vi "MARS Scan Data Analysis Wrapper.vi"(9 "Ratio Graph in":refnum<vi>, 10 "Listbox":i32[](array[numeric]), 11 "Active Meas.":i32) -> (0 "FoM Graph":dbl[][](array[numeric]), 1 "Fit Histogram":i32[][](array[numeric]), 2 "Ratio Graph":i32[][](array[numeric]), 3 "FoM":dbl, 4 "FoM_2nd_max":dbl, 5 "FoM_1st_max":dbl, 6 "FoM_2nd_min":dbl, 7 "FoM_1st_min":dbl)   [LabVIEW 2015]
uses:
  Data_Analysis_subvis/MARS_Scan_Data_Analysis_global.vi
panel:
  out "2nd period 2":dbl[](array[numeric])
  out "1st period 2":dbl[](array[numeric])
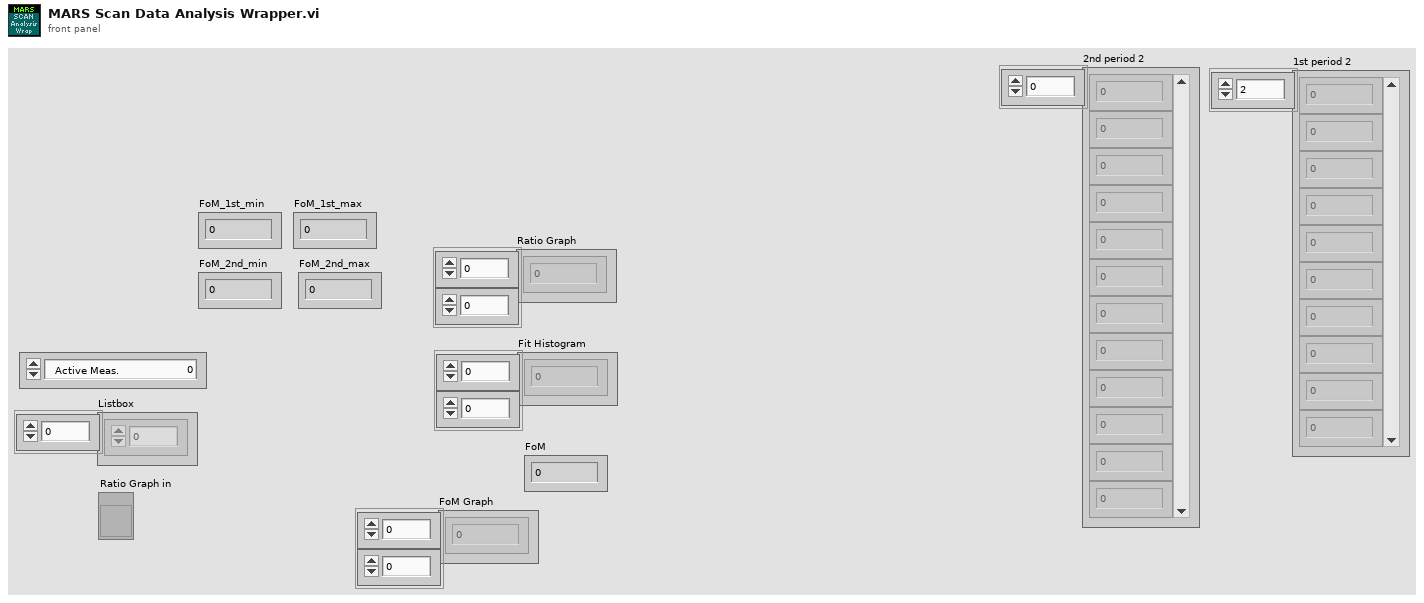
[diagram p1: front panel]
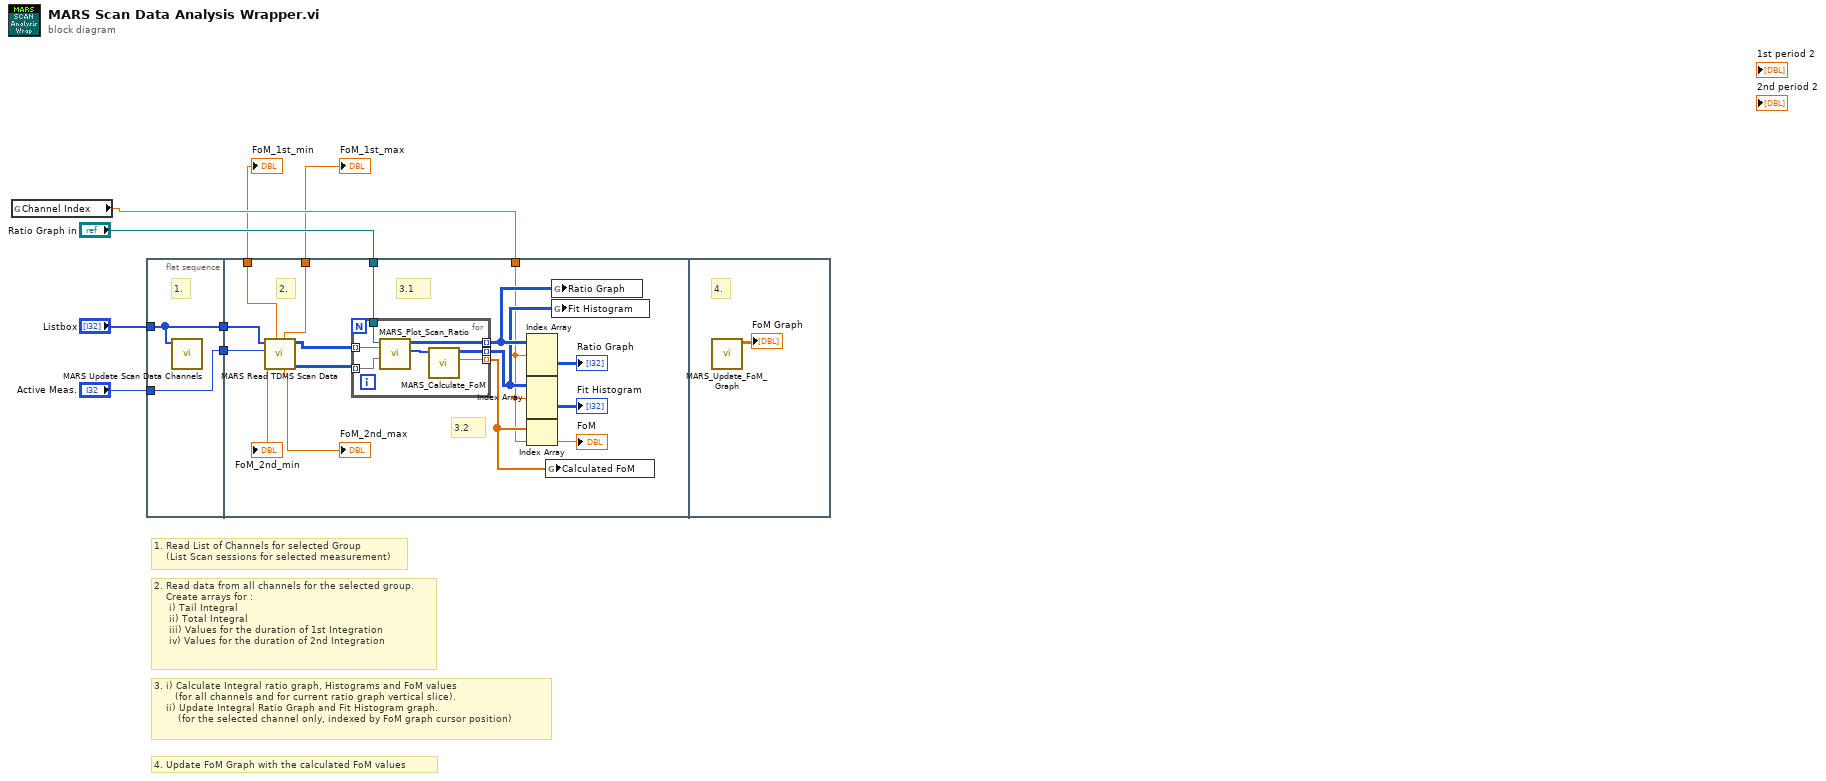
[diagram p0: block diagram]
diagram:
  # "4. Update FoM Graph with the calculated FoM values"
  # "3. i) Calculate Integral ratio graph, Histograms and FoM values\n       (for all channels and for current ratio graph vertical slice).\n    ii) Update Integral Ratio Graph and Fit Histogram graph.\n        (for the selected channel only, indexed by FoM graph cursor position)"
  # "2. Read data from all channels for the selected group.\n    Create arrays for : \n     i) Tail Integral\n     ii) Total Integral\n     iii) Values for the duration of 1st Integration\n     iv) Values for the duration of 2nd Integration"
  # "1. Read List of Channels for selected Group\n    (List Scan sessions for selected measurement)"
  n1 = global read "MARS_Scan_Data_Analysis_global.vi" "Channel Index"() -> (w3:dbl)
  n2 = flat-sequence {
    tunnel: "Listbox" -> [w10]
    tunnel: "Active Meas." -> [w9]
    tunnel: [w10] -> w5
    tunnel: [w9] -> w4
    tunnel: "Ratio Graph in" -> [w26]
    tunnel: w3 -> [w15]
    tunnel: w5 -> [w18]
    tunnel: w4 -> [w17]
    tunnel: [w14] -> w2
    tunnel: [w13] -> w1
    frame #0 {
      # "1."
      n3 = call "MARS Update Scan Data Channels.vi"("Listbox"=w10) -> ()  [unwired: 11 in]
    }
    frame #1 {
      # "3.2"
      # "2."
      # "3.1"
      n4 = call "MARS Read TDMS Scan Data.vi"("Active Meas."=w17, "Listbox"=w18) -> ("Scan Total Int"=w19:i32[][], "Scan Tail Int"=w20:i32[][], "FoM_2nd_max"=→"FoM_2nd_max":dbl, "FoM_1st_max"=w14:dbl, "FoM_2nd_min"=→"FoM_2nd_min":dbl, "FoM_1st_min"=w13:dbl)  [unwired: 4 in]
      n5 = for {
        tunnel: w20 -> [w33] mode=indexing
        tunnel: w19 -> [w32] mode=indexing
        tunnel: [w31] -> w22 mode=indexing
        tunnel: [w29] -> w21 mode=indexing
        tunnel: [w28] -> w16 mode=indexing
        tunnel: w26 -> [w27]
        n6 = call "MARS_Plot_Scan_Ratio.vi"("Total Integral"=w32, "Tail Integral in"=w33, "IntensityGraph in"=w27) -> ("Histogram"=w30:i32[], "Ratio Graph"=w31:i32[][])  [unwired: 7 in]
        n7 = call "MARS_Calculate_FoM.vi"("Histogram"=w30) -> ("FoM"=w28:dbl, "Fit Histogram"=w29:i32[][])  [unwired: 7 in, 2 out]
      }
      n8 = Index Array(array=w22, index (dim 0)=w15) -> (element=→"Ratio Graph":i32[][])  [unwired: 2 in]
      n9 = Index Array(array=w21, index (dim 0)=w15) -> (element=→"Fit Histogram":i32[][])  [unwired: 2 in]
      n10 = Index Array(array=w16, index=w15) -> (element=→"FoM":dbl)
      n11 = global write "MARS_Scan_Data_Analysis_global.vi" "Calculated FoM"(w16) -> ()
      n12 = global write "MARS_Scan_Data_Analysis_global.vi" "Ratio Graph"(w22) -> ()
      n13 = global write "MARS_Scan_Data_Analysis_global.vi" "Fit Histogram"(w21) -> ()
    }
    frame #2 {
      # "4."
      n14 = call "MARS_Update_FoM_Graph.vi"() -> ("FoM Graph"=→"FoM Graph":dbl[][])  [unwired: 11 in]
    }
  }
  "FoM_1st_max" <- w2
  "FoM_1st_min" <- w1
